vi "Calculate_Cooridanets_Of_Joints.vi"(8 "error in (no error)":errorcluster, 11 "reference in":refnum<class "Manipulator.lvclass">) -> (0 "error out":errorcluster, 3 "reference out":refnum<class "Manipulator.lvclass">)   [LabVIEW 2014, in "Manipulator.lvclass"]
uses:
  Manipulator.lvclass
panel:
  out "Angles":T1
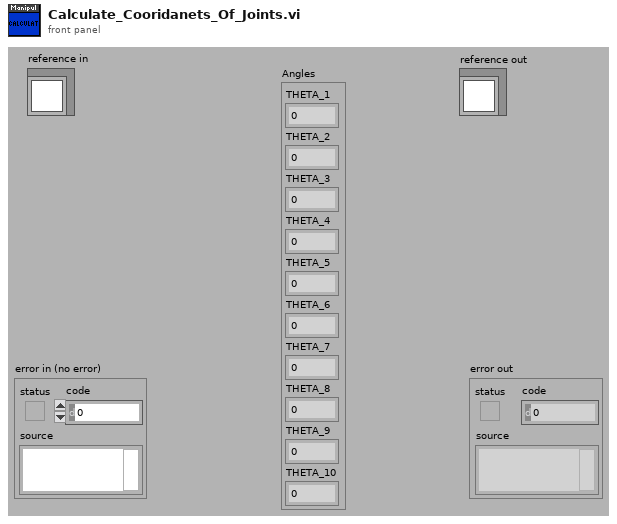
[diagram p1: front panel]
types:
  T1 = cluster{"THETA_1":dbl, "THETA_2":dbl, "THETA_3":dbl, "THETA_4":dbl, "THETA_5":dbl, "THETA_6":dbl, "THETA_7":dbl, "THETA_8":dbl, "THETA_9":dbl, "THETA_10":dbl}
  T2 = typedef "Manipulator.lvclass/ObjectAttributes.ctl" = cluster{"Coordinates":cluster{"X":dbl, "Y":dbl, "Z":dbl}, "Angles":cluster{"THETA_1":dbl, "THETA_2":dbl, "THETA_3":dbl, "THETA_4":dbl, "THETA_5":dbl, "THETA_6":dbl, "THETA_7":dbl, "THETA_8":dbl, "THETA_9":dbl, "THETA_10":dbl}, "Lengths":cluster{"a":dbl, "b":dbl, "c":dbl, "d":dbl, "e":dbl}, "Coordinates of joints":cluster{"A":cluster{"X":dbl, "Y":dbl, "Z":dbl}, "B":cluster{"X":dbl, "Y":dbl, "Z":dbl}, "C":cluster{"X":dbl, "Y":dbl, "Z":dbl}, "D":cluster{"X":dbl, "Y":dbl, "Z":dbl}}}
  T3 = cluster{" OUT (DEG)":dbl, " OUT (DEG)":dbl, " OUT (DEG)":dbl, " OUT (DEG)":dbl, " OUT (DEG)":dbl, " OUT (DEG)":dbl, " OUT (DEG)":dbl, " OUT (DEG)":dbl, " OUT (DEG)":dbl, " OUT (DEG)":dbl}
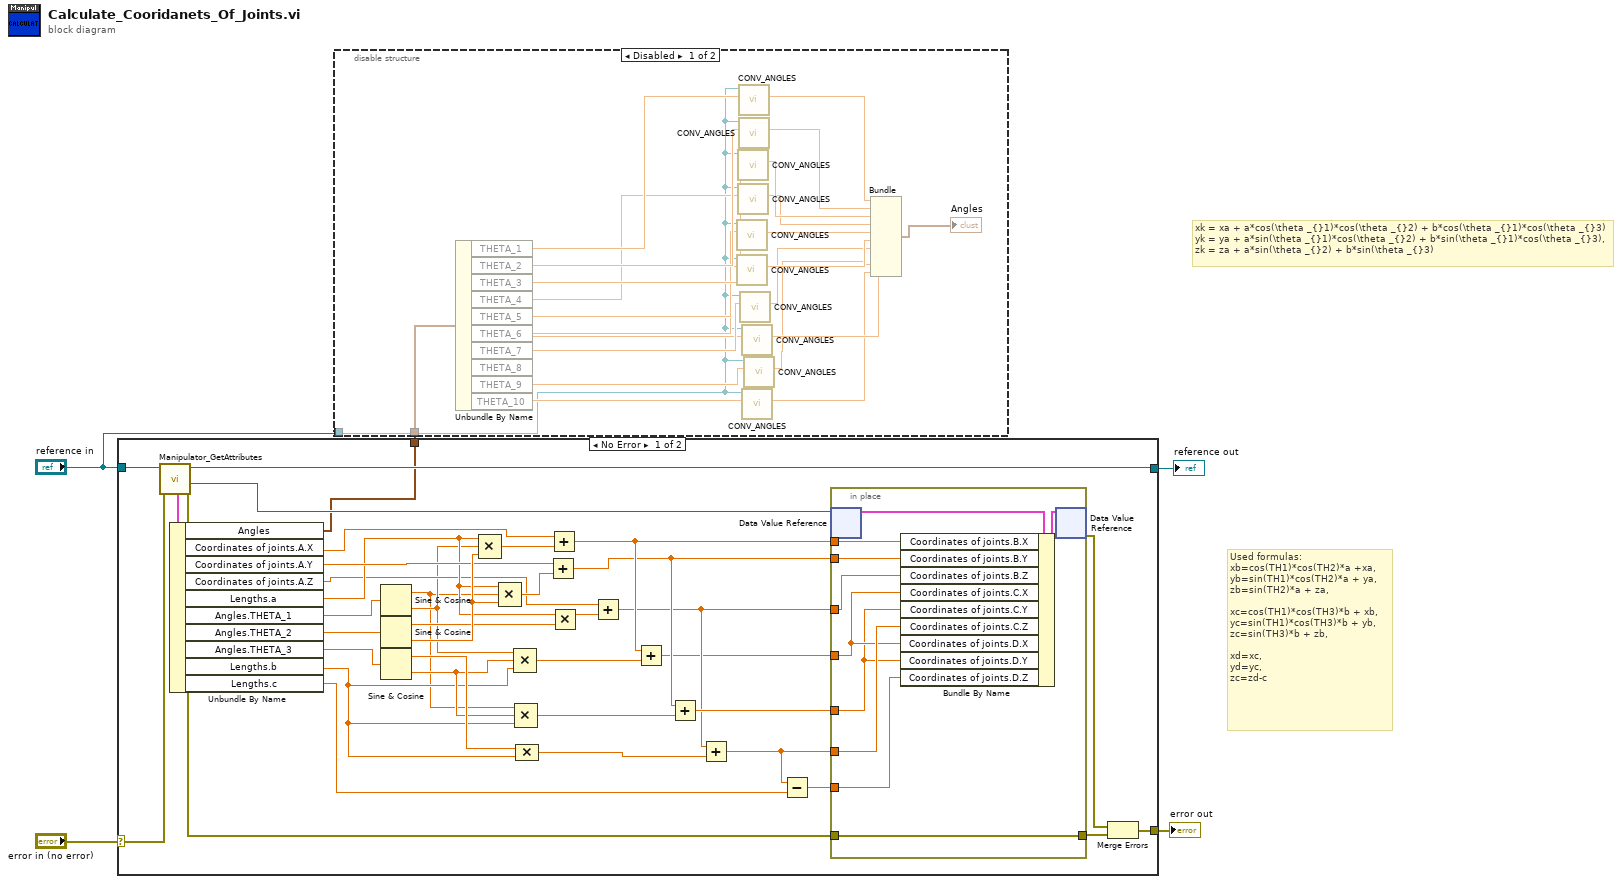
[diagram p0: block diagram]
diagram:
  # "xk = xa + a*cos(\\theta _{}1)*cos(\\theta _{}2) + b*cos(\\theta _{}1)*cos(\\theta _{}3)\nyk = ya + a*sin(\\theta _{}1)*cos(\\theta _{}2) + b*sin(\\theta _{}1)*cos(\\theta _{}3),\nzk = za + a*sin(\\theta _{}2) + b*sin(\\theta _{}3)"
  # "Used formulas:\nxb=cos(TH1)*cos(TH2)*a +xa,\nyb=sin(TH1)*cos(TH2)*a + ya,\nzb=sin(TH2)*a + za,\n\nxc=cos(TH1)*cos(TH3)*b + xb,\nyc=sin(TH1)*cos(TH3)*b + yb,\nzc=sin(TH3)*b + zb,\n\nxd=xc,\nyd=yc,\nzc=zd-c"
  n1 = case shown="No Error" "error in (no error)" {
    selector: "error in (no error)" -> [w42 w55]
    tunnel: [w12 w55] -> w3
    tunnel: [w40 w54] -> w4
    tunnel: "reference in" -> [w43 w54]
    tunnel: [w9 _] -> w2
    frame No Error {
      n2 = call "Manipulator_GetAttributes.vi"("error in (no error)"=w42, "reference in"=w43) -> ("error out"=w38:errorcluster, "DataRef"=w39:refnum<data-value>, "Data"=w41:T2, "reference out"=w40:refnum<class "Manipulator.lvclass">)  [unwired: 6 in]
      n3 = Unbundle By Name(w41) -> ("Angles"=w9:T1, "Coordinates of joints.A.X"=w34:dbl, "Coordinates of joints.A.Y"=w30:dbl, "Coordinates of joints.A.Z"=w26:dbl, "Lengths.a"=w28:dbl, "Angles.THETA_1"=w37:dbl, "Angles.THETA_2"=w36:dbl, "Angles.THETA_3"=w35:dbl, "Lengths.b"=w18:dbl, "Lengths.c"=w14:dbl)
      n4 = Sine & Cosine(0:w37) -> (1:w7:dbl, 2:w8:dbl)
      n5 = Sine & Cosine(0:w36) -> (1:w29:dbl, 2:w32:dbl)
      n6 = Sine & Cosine(0:w35) -> (1:w20:dbl, 2:w19:dbl)
      n7 = Compound Arithmetic op=MULTIPLY(w28, w8, w32) -> (w33:dbl)
      n8 = Compound Arithmetic op=MULTIPLY(w28, w7, w32) -> (w31:dbl)
      n9 = Compound Arithmetic op=MULTIPLY(w8, w19, w18) -> (w24:dbl)
      n10 = Compound Arithmetic op=MULTIPLY(w7, w19, w18) -> (w22:dbl)
      n11 = Compound Arithmetic op=MULTIPLY(w20, w18) -> (w16:dbl)
      n12 = Add(x=w30, y=w31) -> (x+y=w23:dbl)
      n13 = Add(x=w34, y=w33) -> (x+y=w25:dbl)
      n14 = Multiply(x=w28, y=w29) -> (x*y=w27:dbl)
      n15 = Add(x=w26, y=w27) -> (x+y=w17:dbl)
      n16 = Add(x=w25, y=w24) -> (x+y=w6:dbl)
      n17 = Add(x=w23, y=w22) -> (x+y=w21:dbl)
      n18 = Add(x=w17, y=w16) -> (x+y=w15:dbl)
      n19 = Subtract(x=w15, y=w14) -> (x-y=w13:dbl)
      n20 = in-place {
        in-place-border: w38 -> [w52]
        in-place-border: [w52] -> w11
        in-place-border: w25 -> [w50]
        in-place-border: w23 -> [w49]
        in-place-border: w17 -> [w48]
        in-place-border: w6 -> [w46]
        in-place-border: w21 -> [w45]
        in-place-border: w15 -> [w47]
        in-place-border: w13 -> [w44]
        n21 = in-place-dvr #1(w39) -> (w51:T2)  [unwired: 1 out]
        n22 = Bundle By Name(cluster=w51, "Coordinates of joints.B.X"=w50, "Coordinates of joints.B.Y"=w49, "Coordinates of joints.B.Z"=w48, "Coordinates of joints.C.X"=w46, "Coordinates of joints.C.Y"=w45, "Coordinates of joints.C.Z"=w47, "Coordinates of joints.D.X"=w46, "Coordinates of joints.D.Y"=w45, "Coordinates of joints.D.Z"=w44) -> (w53:T2)
        n23 = in-place-dvr #1(w53) -> (w10:errorcluster)  [unwired: 1 out]
      }
      n24 = Merge Errors(w10, w11) -> (w12:errorcluster)
    }
    frame Error {
    }
  }
  "error out" <- w3
  "reference out" <- w4
  n25 = disable-structure shown="Disabled" {
    disable-tunnel: w2 -> [w78 _]
    disable-tunnel: "reference in" -> [w56 _]
    frame Disabled {
      n26 = Unbundle By Name(w78) -> ("THETA_1"=w77:dbl, "THETA_2"=w76:dbl, "THETA_3"=w75:dbl, "THETA_4"=w74:dbl, "THETA_5"=w73:dbl, "THETA_6"=w72:dbl, "THETA_7"=w71:dbl, "THETA_8"=w70:dbl, "THETA_9"=w69:dbl, "THETA_10"=w68:dbl)
      n27 = call "CONV_ANGLES.vi"("IN (RAD)"=w73, "reference in"=w56) -> ("OUT (DEG)"=w63:dbl)  [unwired: 6 in, 3 out]
      n28 = call "CONV_ANGLES.vi"("IN (RAD)"=w72, "reference in"=w56) -> ("OUT (DEG)"=w62:dbl)  [unwired: 6 in, 3 out]
      n29 = call "CONV_ANGLES.vi"("IN (RAD)"=w75, "reference in"=w56) -> ("OUT (DEG)"=w65:dbl)  [unwired: 6 in, 3 out]
      n30 = call "CONV_ANGLES.vi"("IN (RAD)"=w74, "reference in"=w56) -> ("OUT (DEG)"=w64:dbl)  [unwired: 6 in, 3 out]
      n31 = call "CONV_ANGLES.vi"("IN (RAD)"=w77, "reference in"=w56) -> ("OUT (DEG)"=w67:dbl)  [unwired: 6 in, 3 out]
      n32 = call "CONV_ANGLES.vi"("IN (RAD)"=w76, "reference in"=w56) -> ("OUT (DEG)"=w66:dbl)  [unwired: 6 in, 3 out]
      n33 = call "CONV_ANGLES.vi"("IN (RAD)"=w71, "reference in"=w56) -> ("OUT (DEG)"=w61:dbl)  [unwired: 6 in, 3 out]
      n34 = call "CONV_ANGLES.vi"("IN (RAD)"=w70, "reference in"=w56) -> ("OUT (DEG)"=w60:dbl)  [unwired: 6 in, 3 out]
      n35 = call "CONV_ANGLES.vi"("IN (RAD)"=w68, "reference in"=w56) -> ("OUT (DEG)"=w58:dbl)  [unwired: 6 in, 3 out]
      n36 = call "CONV_ANGLES.vi"("IN (RAD)"=w69, "reference in"=w56) -> ("OUT (DEG)"=w59:dbl)  [unwired: 6 in, 3 out]
      n37 = Bundle("OUT (DEG)"=w67, "OUT (DEG)"=w66, "OUT (DEG)"=w65, "OUT (DEG)"=w64, "OUT (DEG)"=w63, "OUT (DEG)"=w62, "OUT (DEG)"=w61, "OUT (DEG)"=w60, "OUT (DEG)"=w59, "OUT (DEG)"=w58) -> (→"Angles":T3)  [unwired: 1 in]
    }
    frame Enabled {
    }
  }
